vi "Bug globals.vi"() -> ()   [LabVIEW 2019]
doc: "Thise are the global variables for the bug C(T) experiment.\n\nPaul K Dxion\nP3600\nCSUSB Physics"
uses:
  typedefs/temp cont cluster.ctl
  typedefs/temp exec cluster.ctl
  typedefs/temp mode enum.ctl
  typedefs/temp indicator.ctl
  typedefs/temp control status.ctl
  typedefs/PID control parameters.ctl
  typedefs/temp cont utility.ctl
  typedefs/measurement.ctl
  typedefs/wvfm acq params.ctl
  typedefs/result.ctl
  typedefs/cap fit params.ctl
panel:
  out "imm meas":bool
  in  "results":T1[](array[typedef])
  in  "meas":T3={"wvfm params"={"Num of avg"=100, "Num points"=1000, "Meas rate (Hz)"=100000.0}, "avg"={"t0"=timestamp(0 s since 1904-01-01), "dt"=1.0, "Y"=[]}, "raw wvfms"=[], "progress"={"avg done"=FALSE, "meas index"=0, "N waves"=0}, "t (s)"=0.0}
  out "x":bool
  in  "temp":T5={"T exec"={"T mode"=enum."Exit", "exec setpoint"=30.0, "reset"=FALSE, "man power"=0.5, "man"=FALSE, "log"=FALSE, "clear"=FALSE}, "T status"={"Control status"=enum."Below Control Band", "Temp"=0.0, "Power"=0.0, "Time in settle band"=0.0, "Settled"=FALSE, "Low"=FALSE, "High"=FALSE, "Setpoint"=30.0, "Control"=FALSE, "In Settle Band"=FALSE}, "T params"={"Setpoint"=30.0, "Control Bandwidth"=4.0, "Integral Time"=30.0, "Int\nON"=TRUE, "Derivative Tme"=0.5, "Der\nON"=TRUE, "Settle Bandwidth"=1.0, "Settle Time"=60.0}, "utility"={"meas index"=0, "wait (ms)"=300, "H Vmax"=8.5, "power out"=0.0, "heat volt out"=0.0, "heat volt in"=0.0, "therm volt"=0.0, "t T P hist"=[], "cont hist"=[]}} {"utility"."therm volt" format="%_6g"; "utility"."heat volt in" format="%_6g"; "utility"."heat volt out" format="%_6g"; "utility"."power out" format="%_6g"; "utility"."H Vmax" format="%_6g"; "T exec"."man power" format="%_6g"; "T exec"."exec setpoint" format="%_6g"; "T params"."Settle Time" step=1.0; "T params"."Settle Bandwidth" step=0.01; "T params"."Derivative Tme" step=0.01; "T params"."Integral Time" step=1.0; "T params"."Control Bandwidth" step=0.1; "T params"."Setpoint" step=0.1; "T status"."Setpoint" format="%_6g"; "T status"."Power" format="%_6g"; "T status"."Temp" format="%_6g"}
  # "exec, wait, and T params are under exec control"
  # "wave params are under exec control"
  # "T status and the voltages are under DAQ state machine control"
  # "all others under DAQ state machine control"
  # "under exec control"
  # "main global stop used for loops where locals cant get"
  # "bypasses the\nsettle for wait\nfeature"
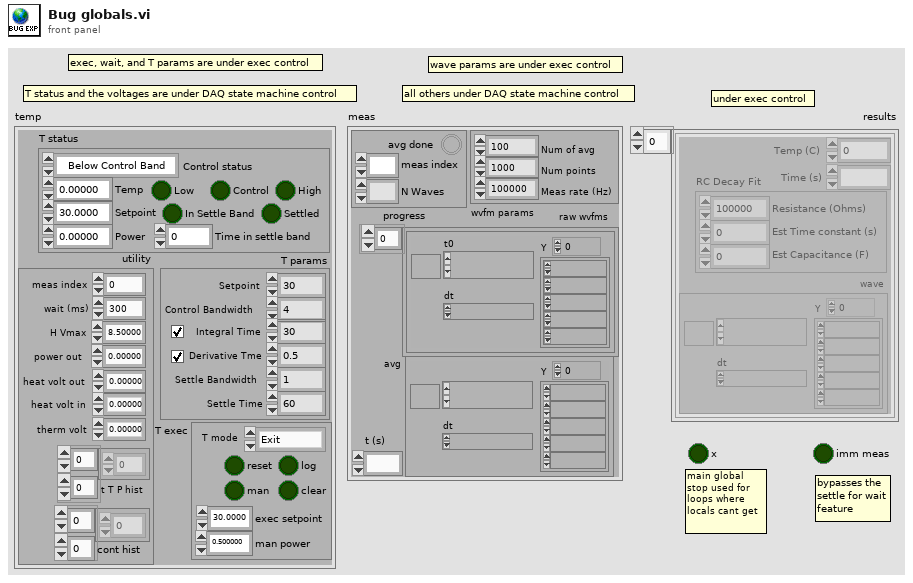
[diagram p1: front panel]
types:
  T1 = typedef "result.ctl" = cluster{"Temp (C)":dbl, "RC Fit":T2, "wave":waveform(dbl), "Time (s)":dbl}
  T2 = typedef "cap fit params.ctl" = cluster{"Resistance (Ohms)":dbl, "Est Time constant (s)":dbl, "Est Capacitance (F)":dbl}
  T3 = typedef "measurement.ctl" = cluster{"wvfm params":T4, "avg":waveform(dbl), "raw wvfms":waveform(dbl)[], "progress":cluster{"avg done":bool, "meas index":i32, "N waves":i32}, "t (s)":dbl}
  T4 = typedef "wvfm acq params.ctl" = cluster{"Num of avg":i32, "Num points":i32, "Meas rate (Hz)":dbl}
  T5 = typedef "temp cont cluster.ctl" = cluster{"T exec":T6, "T status":T8, "T params":T10, "utility":T11}
  T6 = typedef "temp exec cluster.ctl" = cluster{"T mode":T7, "exec setpoint":dbl, "reset":bool, "man power":dbl, "man":bool, "log":bool, "clear":bool}
  T7 = typedef "temp mode enum.ctl" = enum16{"settling", "measuring", "holding", "Exit"}
  T8 = typedef "temp indicator.ctl" = cluster{"Control status":T9, "Temp":dbl, "Power":dbl, "Time in settle band":dbl, "Settled":bool, "Low":bool, "High":bool, "Setpoint":dbl, "Control":bool, "In Settle Band":bool}
  T9 = typedef "temp control status.ctl" = enum16{"In Settle Band", "In Control Band", "Below Control Band", "Above Control Band"}
  T10 = typedef "PID control parameters.ctl" = cluster{"Setpoint":dbl, "Control Bandwidth":dbl, "Integral Time":dbl, "Int\nON":bool, "Derivative Tme":dbl, "Der\nON":bool, "Settle Bandwidth":dbl, "Settle Time":dbl}
  T11 = typedef "temp cont utility.ctl" = cluster{"meas index":i32, "wait (ms)":i32, "H Vmax":dbl, "power out":dbl, "heat volt out":dbl, "heat volt in":dbl, "therm volt":dbl, "t T P hist":dbl[][], "cont hist":dbl[][]}
diagram:
